vi "JetCU User Interface.vi"() -> ()   [LabVIEW 2017]
panel:
  out "ECU VISA Out":refnum<visa-resource-name>
  in  "ECU VISA In":refnum<visa-resource-name>
  out "Error Out":errorcluster
  in  "Error In":errorcluster
  out "Read Buffer":string
  in  "Command In":string
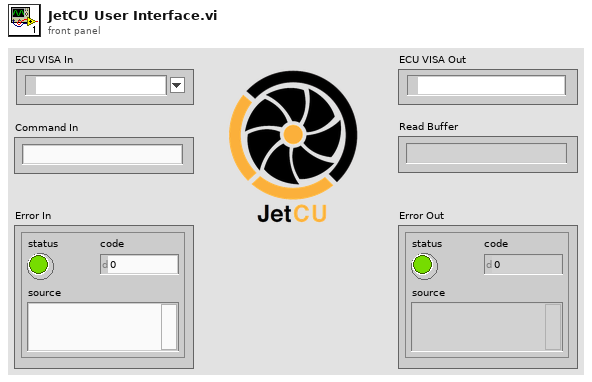
[diagram p1: front panel]
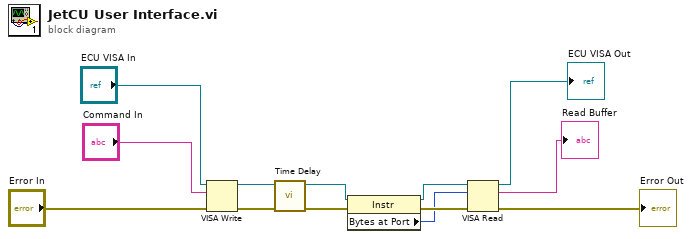
[diagram p0: block diagram]
diagram:
  n1 = VISA Write(VISA resource name="ECU VISA In", write buffer="Command In", error in (no error)="Error In") -> (VISA resource name out=w3:refnum<visa-resource-name>, error out=w11:errorcluster)  [unwired: 1 out]
  n2 = call "Time Delay"("error in (no error)"=w11) -> ("error out"=w5:errorcluster)  [unwired: 10 in]
  n3 = property class="Instr"(reference=w3, error in=w5) -> (reference out=w2:refnum<visa-resource-name>, error out=w4:errorcluster, "Bytes at Port"=w1:u32)
  n4 = VISA Read(VISA resource name=w2, byte count=w1, error in (no error)=w4) -> (VISA resource name out=→"ECU VISA Out":refnum<visa-resource-name>, read buffer=→"Read Buffer":string, error out=→"Error Out":errorcluster)  [unwired: 1 out]
